vi "Graphviz Path.vi"(8 "error in":errorcluster) -> (0 "error out":errorcluster, 3 "Graphviz Path":path)   [LabVIEW 2020, in "SimpleDependencyInspector.lvlib"]
uses:
  SimpleDependencyInspector.lvlib
  <vilib>/Utility/sysdir.llb/System Directory Type.ctl
  Module Name--constant.vi
  <vilib>/Utility/error.llb/Error Cluster From Error Code.vi
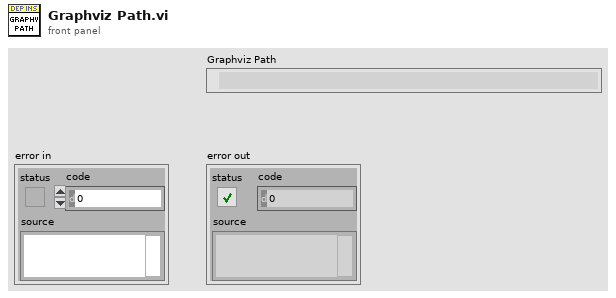
[diagram p1: front panel]
types:
  T1 = typedef "System Directory Type.ctl" = i32
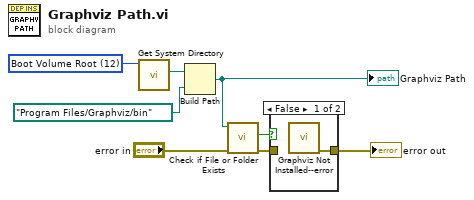
[diagram p0: block diagram]
diagram:
  w5 = T1 12 items=["User Home"=0, "User Desktop"=1, "User Documents"=2, "User Application Data"=3, "User Preferences"=4, "User Temporary"=5, "Public Documents"=6, "Public Application Data"=7, "Public Preferences"=8, "Public Cache"=13, "System Core Libraries"=9, "System Installed Libraries"=10, "Application Files"=11, "Boot Volume Root"=12] ("system directory type")
  n1 = call <vilib>:"Get System Directory.vi"("system directory type"=w5) -> ("system directory"=w4:path)  [unwired: 10 in]
  n2 = Build Path(base path=w4, name or relative path=path "Program Files/Graphviz/bin") -> (appended path=w2:path)
  "Graphviz Path" <- w2
  n3 = call <vilib>:"Check if File or Folder Exists.vi"("error in (no error)"="error in", "path"=w2) -> ("error out"=w7:errorcluster, "file or folder exists?"=w1:bool)  [unwired: 7 in, 1 out]
  n4 = case shown="False" w1 {
    tunnel: [w9 w10] -> w8
    tunnel: w7 -> [_ w10]
    frame False {
      n5 = call "Graphviz Not Installed--error.vi"() -> ("error out"=w9:errorcluster)  [unwired: 11 in]
    }
    frame True {
    }
  }
  "error out" <- w8
